vi "LS330_STATUS.vi"(8 "error in (no error)":errorcluster, 11 "VISA Refnum in":refnum<visa-resource-name>) -> (0 "error out":errorcluster, 2 "Status":cluster{T1, T1}, 3 "VISA resource name out":refnum<visa-resource-name>)   [LabVIEW 2021]
uses:
  LS330_Status_Bundle.ctl
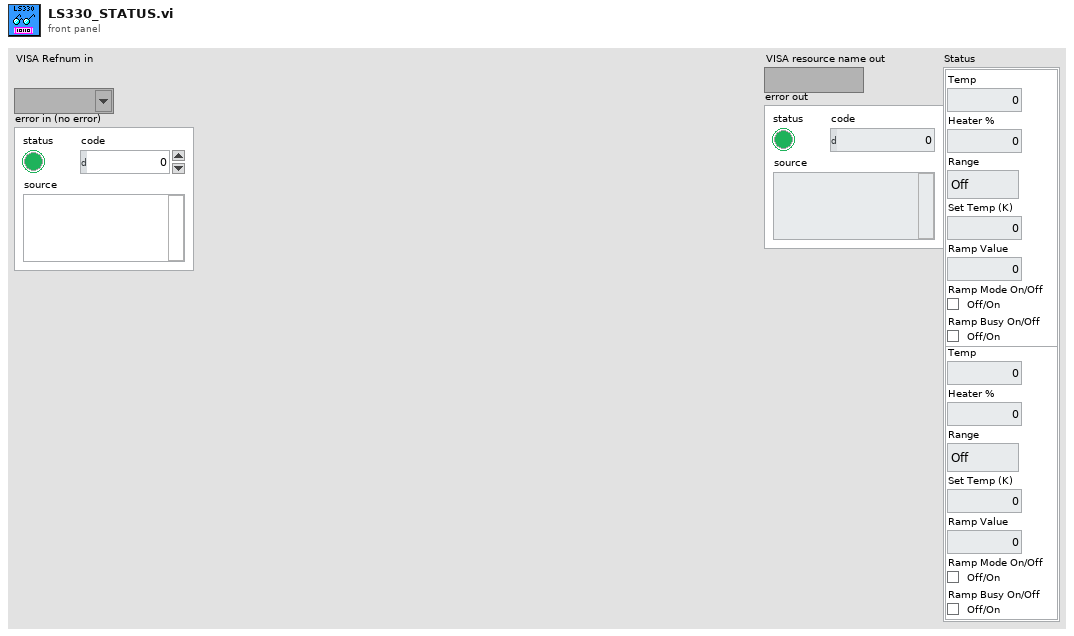
[diagram p1: front panel]
types:
  T1 = typedef "LS330_Status_Bundle.ctl" = cluster{"Temp":dbl, "Heater %":dbl, "Range":enum16{"Off", "Low", "Medium", "High"}, "Set Temp (K)":dbl, "Ramp Value":dbl, "Ramp Mode On/Off":bool, "Ramp Busy On/Off":bool}
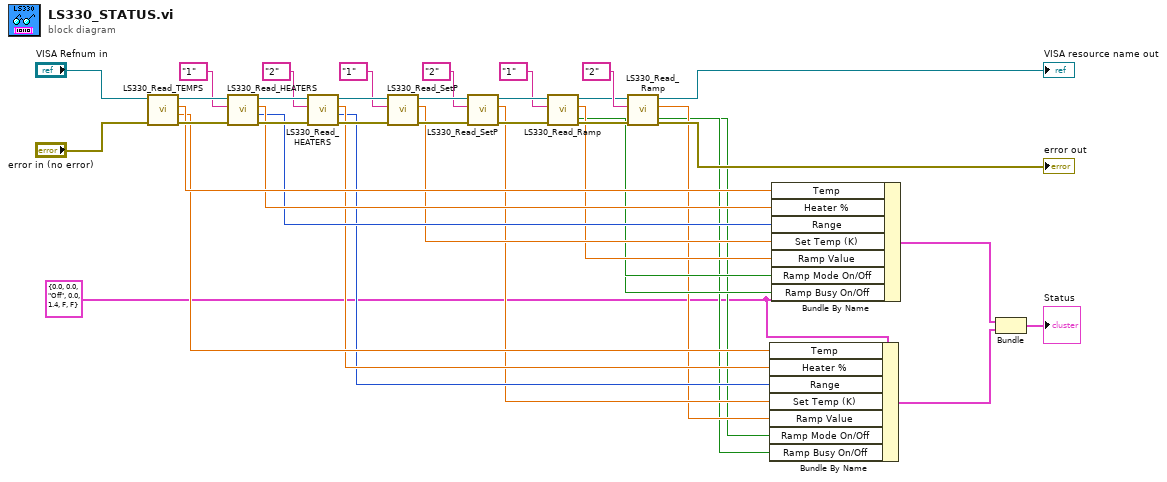
[diagram p0: block diagram]
diagram:
  w2 = T1 {"Temp"=0.0, "Heater %"=0.0, "Range"=enum."Off", "Set Temp (K)"=0.0, "Ramp Value"=1.4, "Ramp Mode On/Off"=FALSE, "Ramp Busy On/Off"=FALSE}
  n1 = call "LS330_Read_TEMPS.vi"("error in (no error)"="error in (no error)", "VISA Refnum in"="VISA Refnum in") -> ("error out"=w37:errorcluster, "Temp B (K)"=w11:dbl, "Temp A (K)"=w18:dbl, "VISA Refnum out"=w38:refnum<visa-resource-name>)  [unwired: 4 in]
  n2 = call "LS330_Read_HEATERS.vi"("error in (no error)"=w37, "Heater"="1", "VISA Refnum in"=w38) -> ("error out"=w35:errorcluster, "Range"=w16:enum16{"Off", "Low", "Medium", "High"}, "Heater %"=w17:dbl, "VISA Refnum out"=w36:refnum<visa-resource-name>)  [unwired: 5 in]
  n3 = call "LS330_Read_HEATERS.vi"("error in (no error)"=w35, "Heater"="2", "VISA Refnum in"=w36) -> ("error out"=w31:errorcluster, "Range"=w9:enum16{"Off", "Low", "Medium", "High"}, "Heater %"=w10:dbl, "VISA Refnum out"=w32:refnum<visa-resource-name>)  [unwired: 5 in]
  n4 = call "LS330_Read_SetP.vi"("error in"=w31, "Heater"="1", "VISA resource name"=w32) -> ("error out"=w28:errorcluster, "Set Temp (K)"=w15:dbl, "VISA resource name out"=w29:refnum<visa-resource-name>)  [unwired: 6 in]
  n5 = call "LS330_Read_SetP.vi"("error in"=w28, "Heater"="2", "VISA resource name"=w29) -> ("error out"=w25:errorcluster, "Set Temp (K)"=w8:dbl, "VISA resource name out"=w26:refnum<visa-resource-name>)  [unwired: 6 in]
  n6 = call "LS330_Read_Ramp.vi"("error in"=w25, "Heater"="1", "VISA resource name"=w26) -> ("error out"=w21:errorcluster, "Ramp Value"=w14:dbl, "VISA resource name out"=w22:refnum<visa-resource-name>, "Ramp Mode On/Off"=w13:bool, "Ramp Busy On/Off"=w12:bool)  [unwired: 4 in]
  n7 = call "LS330_Read_Ramp.vi"("error in"=w21, "Heater"="2", "VISA resource name"=w22) -> ("error out"=→"error out":errorcluster, "Ramp Value"=w7:dbl, "VISA resource name out"=→"VISA resource name out":refnum<visa-resource-name>, "Ramp Mode On/Off"=w5:bool, "Ramp Busy On/Off"=w6:bool)  [unwired: 4 in]
  n8 = Bundle By Name(cluster=w2, "Temp"=w11, "Heater %"=w10, "Range"=w9, "Set Temp (K)"=w8, "Ramp Value"=w7, "Ramp Mode On/Off"=w5, "Ramp Busy On/Off"=w6) -> (w3:T1)
  n9 = Bundle By Name(cluster=w2, "Temp"=w18, "Heater %"=w17, "Range"=w16, "Set Temp (K)"=w15, "Ramp Value"=w14, "Ramp Mode On/Off"=w13, "Ramp Busy On/Off"=w12) -> (w4:T1)
  n10 = Bundle(w4, w3) -> (→"Status":cluster{T1, T1})  [unwired: 1 in]
